vi "time interval to time string.vi"(2 "interval scale (ms)":T1, 4 "time interval":u32) -> (1 "Time String":string)   [LabVIEW 2023]
uses:
  interval type.ctl
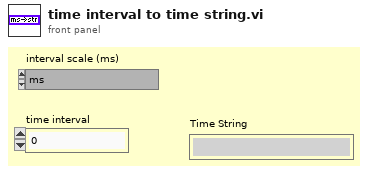
[diagram p1: front panel]
types:
  T1 = typedef "interval type.ctl" = enum16{"ms", "s", "min", "hours", "days", "weeks", "months", "years"}
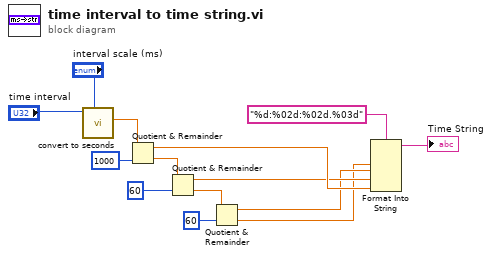
[diagram p0: block diagram]
diagram:
  n1 = call "convert to seconds.vi"("interval scale (s)"="interval scale (ms)", "Value in"="time interval") -> ("ms out"=w1:dbl)  [unwired: 8 in, 1 out]
  n2 = Quotient & Remainder(x=w1, y=u32 1000) -> (x-y*floor(x/y)=w9:dbl, floor(x/y)=w8:dbl)
  n3 = Quotient & Remainder(x=w8, y=u32 60) -> (x-y*floor(x/y)=w7:dbl, floor(x/y)=w6:dbl)
  n4 = Quotient & Remainder(x=w6, y=u32 60) -> (x-y*floor(x/y)=w5:dbl, floor(x/y)=w4:dbl)
  n5 = Format Into String(format string="%d:%02d:%02d.%03d" ("Format String"), w4, w5, w7, w9) -> (resulting string=→"Time String":string)  [unwired: 2 in, 1 out]
